vi "PhotonPNPResult_unpack_OLD.vi"(9 "StartByte":i32, 11 "RawData":u8[](array[numeric])) -> (1 "NextByte":i32, 3 "PNP_Result":T1={"IsPresent"=FALSE, "bestReprojErr"=0.0, "altReprojErr"=0.0, "ambiguity"=0.0, "Best"={"TRANSLATION3D"={"X"=0.0, "Y"=0.0, "Z"=0.0}, "ROTATION3D"={"Q_quaternion"={"R"=1.0, "V"=[0.0, 0.0, 0.0]}}, "XF"=FALSE}, "Alt"={"TRANSLATION3D"={"X"=0.0, "Y"=0.0, "Z"=0.0}, "ROTATION3D"={"Q_quaternion"={"R"=1.0, "V"=[0.0, 0.0, 0.0]}}, "XF"=FALSE}} {"Alt"."TRANSLATION3D"."Z" format="%14.3f"; "Alt"."TRANSLATION3D"."Y" format="%14.3f"; "Alt"."TRANSLATION3D"."X" format="%14.3f"; "Best"."TRANSLATION3D"."Z" format="%14.3f"; "Best"."TRANSLATION3D"."Y" format="%14.3f"; "Best"."TRANSLATION3D"."X" format="%14.3f"})   [LabVIEW 2019, in "PhotonVisionLib.lvlib"]
doc: "Internal function to parse the data for each PNP_Result returned by PhotonCamera_GetLatestResult.\n\nInputs:\n - RawData -- Byte array containing the data to parse.\n - StartingByte -- Index into raw data to start parsing. First byte is index 0.\n\nOutputs:\n - PNP_Result -- Parsed PNP_Result cluster."
uses:
  TypeDef/PhotonPNPResultType.ctl
  <vilib>/Rock Robotics/WPI/ThirdParty/JAS_Junk/TrajLib/TypeDef/TRANSFORM3D.ctl
  <vilib>/Rock Robotics/WPI/ThirdParty/JAS_Junk/TrajLib/TypeDef/TRANSLATION3D.ctl
  <vilib>/Rock Robotics/WPI/ThirdParty/JAS_Junk/TrajLib/TypeDef/ROTATION3D.ctl
  <vilib>/Rock Robotics/WPI/ThirdParty/JAS_Junk/TrajLib/TypeDef/QUATERNION.ctl
  <vilib>/Rock Robotics/WPI/ThirdParty/JAS_Junk/TrajLib/VI/Transform3d_Create_Trans3dRot3d.vi
  <vilib>/Rock Robotics/WPI/ThirdParty/JAS_Junk/TrajLib/VI/Translation3d_Create.vi
  <vilib>/Rock Robotics/WPI/ThirdParty/JAS_Junk/TrajLib/VI/Rotation3d_Create_Quaternion.vi
  <vilib>/Rock Robotics/WPI/ThirdParty/JAS_Junk/TrajLib/VI/Quaternion_New.vi
  <vilib>/Rock Robotics/WPI/ThirdParty/JAS_Junk/TrajLib/VI/Quaternion_Normalize.vi
  <vilib>/Rock Robotics/WPI/ThirdParty/JAS_Junk/TrajLib/VI/Quaternion_New_Default.vi
  PhotonVisionLib.lvlib
  <vilib>/Rock Robotics/WPI/ThirdParty/JAS_Junk/TrajLib/Trajectory_Library.lvlib
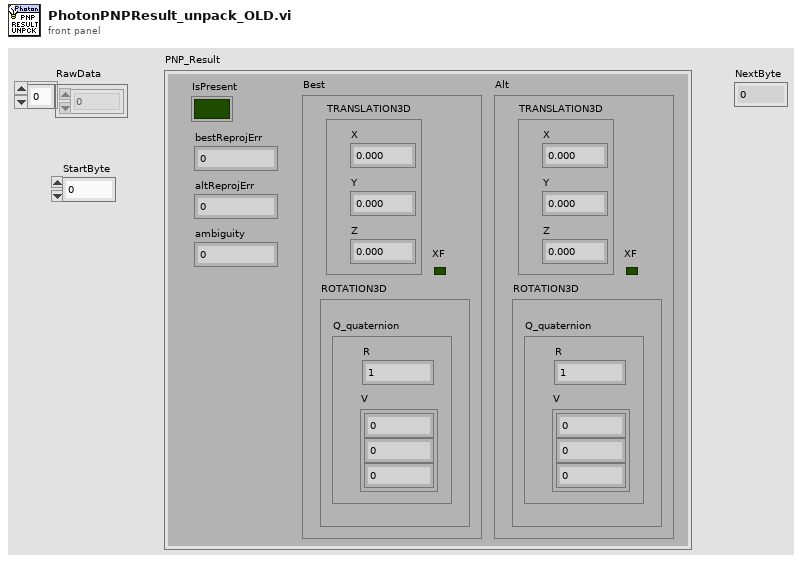
[diagram p1: front panel]
types:
  T1 = typedef "PhotonVisionLib.lvlib/PhotonPNPResultType.ctl" = cluster{"IsPresent":bool, "bestReprojErr":dbl, "altReprojErr":dbl, "ambiguity":dbl, "Best":T2, "Alt":T2}
  T2 = typedef "Trajectory_Library.lvlib/TRANSFORM3D.ctl" = cluster{"TRANSLATION3D":T3, "ROTATION3D":T4, "XF":bool}
  T3 = typedef "Trajectory_Library.lvlib/TRANSLATION3D.ctl" = cluster{"X":dbl, "Y":dbl, "Z":dbl}
  T4 = typedef "Trajectory_Library.lvlib/ROTATION3D.ctl" = cluster{"Q_quaternion":T5}
  T5 = typedef "Trajectory_Library.lvlib/QUATERNION.ctl" = cluster{"R":dbl, "V":dbl[]}
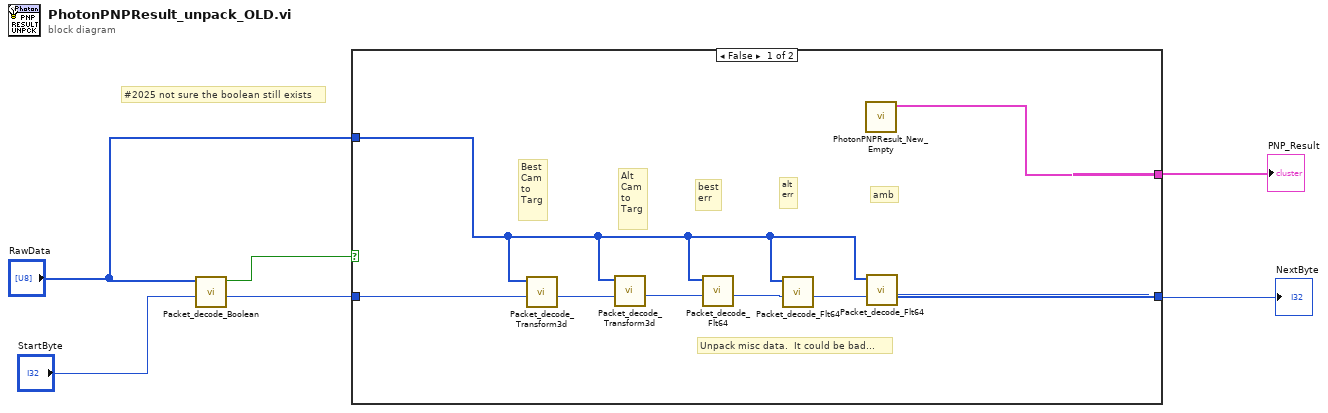
[diagram p0: block diagram]
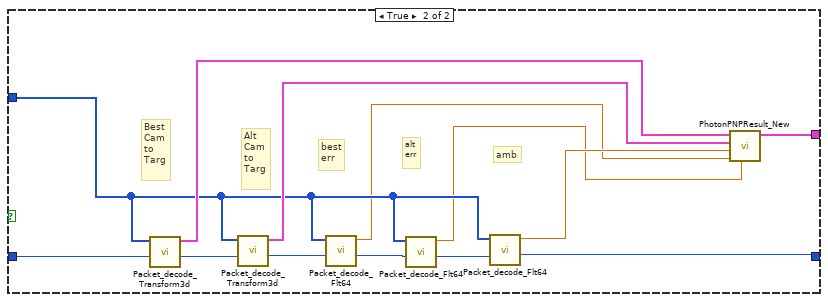
[diagram p2: hidden frame]
diagram:
  # "#2025 not sure the boolean still exists"
  n1 = call "Packet_decode_Boolean.vi"("StartByte"="StartByte", "RawData"="RawData") -> ("NextByte"=w4:i32, "Boolean_Value"=w5:bool)  [unwired: 8 in]
  n2 = case shown="False" w5 {
    tunnel: w4 -> [w8 w25]
    tunnel: [w7 w20] -> w3
    tunnel: [w14 w15] -> w2
    tunnel: "RawData" -> [w9 w19]
    frame False {
      # "Unpack misc data.  It could be bad..."
      # "amb"
      # "alt\nerr"
      # "best\nerr"
      # "Alt\nCam\nto\nTarg"
      # "Best\nCam\nto\nTarg"
      n3 = call "Packet_decode_Transform3d.vi"("NextByte in"=w8, "RawData"=w9) -> ("NextByte out"=w12:i32)  [unwired: 6 in, 1 out]
      n4 = call "Packet_decode_Transform3d.vi"("NextByte in"=w12, "RawData"=w9) -> ("NextByte out"=w13:i32)  [unwired: 6 in, 1 out]
      n5 = call "Packet_decode_Flt64.vi"("StartByte"=w13, "RawData"=w9) -> ("NextByte"=w11:i32)  [unwired: 8 in, 1 out]
      n6 = call "Packet_decode_Flt64.vi"("StartByte"=w11, "RawData"=w9) -> ("NextByte"=w10:i32)  [unwired: 8 in, 1 out]
      n7 = call "PhotonPNPResult_New_Empty.vi"() -> ("PNP_Result"=w14:T1)  [unwired: 11 in]
      n8 = call "Packet_decode_Flt64.vi"("StartByte"=w10, "RawData"=w9) -> ("NextByte"=w7:i32)  [unwired: 8 in, 1 out]
    }
    frame True {
      # "amb"
      # "alt\nerr"
      # "best\nerr"
      # "Alt\nCam\nto\nTarg"
      # "Best\nCam\nto\nTarg"
      n9 = call "Packet_decode_Transform3d.vi"("NextByte in"=w25, "RawData"=w19) -> ("NextByte out"=w26:i32, "Transform3d"=w24:T2)  [unwired: 6 in]
      n10 = call "Packet_decode_Transform3d.vi"("NextByte in"=w26, "RawData"=w19) -> ("NextByte out"=w27:i32, "Transform3d"=w23:T2)  [unwired: 6 in]
      n11 = call "Packet_decode_Flt64.vi"("StartByte"=w27, "RawData"=w19) -> ("NextByte"=w22:i32, "Flt64_Value"=w17:dbl)  [unwired: 8 in]
      n12 = call "Packet_decode_Flt64.vi"("StartByte"=w22, "RawData"=w19) -> ("NextByte"=w21:i32, "Flt64_Value"=w16:dbl)  [unwired: 8 in]
      n13 = call "Packet_decode_Flt64.vi"("StartByte"=w21, "RawData"=w19) -> ("NextByte"=w20:i32, "Flt64_Value"=w18:dbl)  [unwired: 8 in]
      n14 = call "PhotonPNPResult_New.vi"("altReprojErr"=w16, "bestReprojErr"=w17, "ambiguity"=w18, "Alt"=w23, "Best"=w24) -> ("PNP_Result"=w15:T1)  [unwired: 6 in]
    }
  }
  "PNP_Result" <- w2
  "NextByte" <- w3
